vi "Gestion User.vi"(8 "error in (no error)":errorcluster caption="entrée d'erreur (pas d'erreur)", 9 "Fonction":T2(ring), 10 "Commade User":T1) -> (0 "error out":errorcluster caption="sortie d'erreur", 2 "Retour User":T1, 3 "Liste code Operator":string[](array[string]))   [LabVIEW 2020]
uses:
  <vilib>/Utility/config.llb/Config Data RefNum.ctl
  Commande Action Gestion User.ctl
  <vilib>/Utility/config.llb/Read Key (String).vi
  <vilib>/Utility/config.llb/Write Key (String).vi
  <vilib>/Utility/config.llb/NI_LVConfig.lvlib
  Commun VI/Library Commun.lvlib
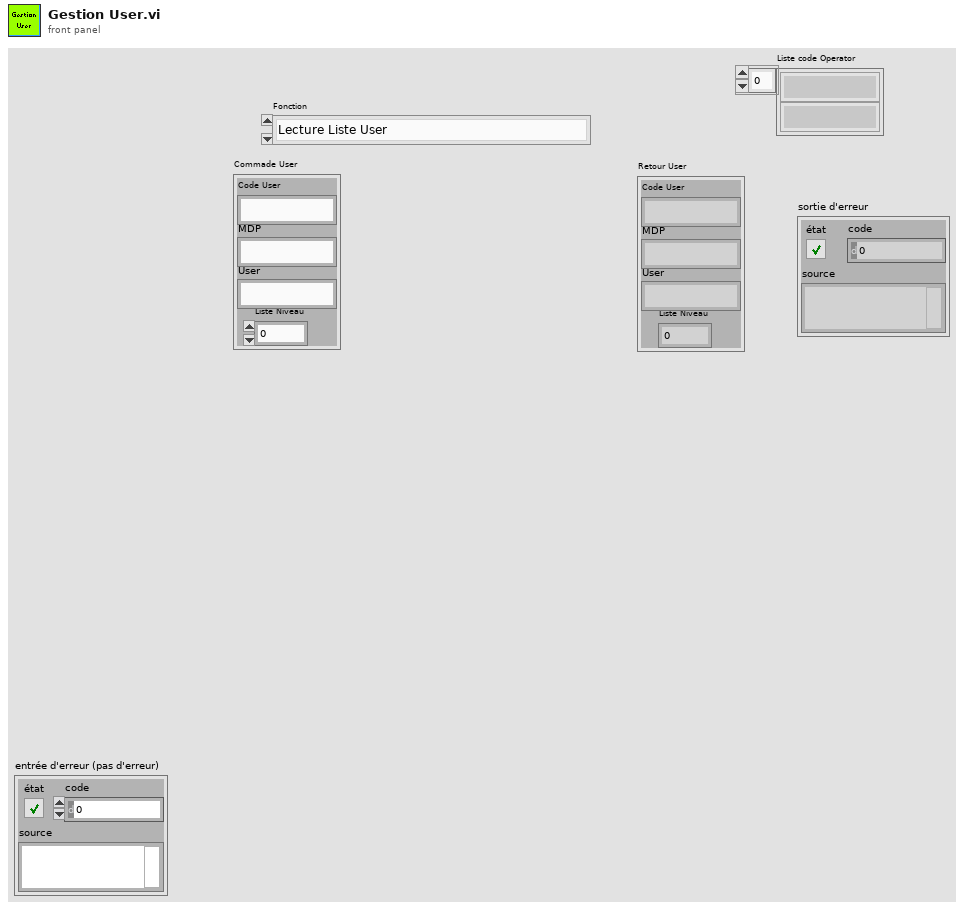
[diagram p1: front panel]
types:
  T1 = cluster{"Code User":string, "MDP":string, "User":string, "Liste Niveau":u16}
  T2 = enum16{"Lecture Liste User", "Lecture User", "Suppression User", "Write User"}
  T3 = cluster{" Section User":string, "Section Grade":string, "Section Password":string}
  T4 = typedef "Commande Action Gestion User.ctl" = enum16{"Ouverture File", "Fermeture File", "Lecture Liste Code User", "Lecture User", "Supression Liste User", "Write User", "Gestion si erreur Decodage"}
  T5 = typedef "NI_LVConfig.lvlib/Config Data RefNum.ctl" = refnum<k1>
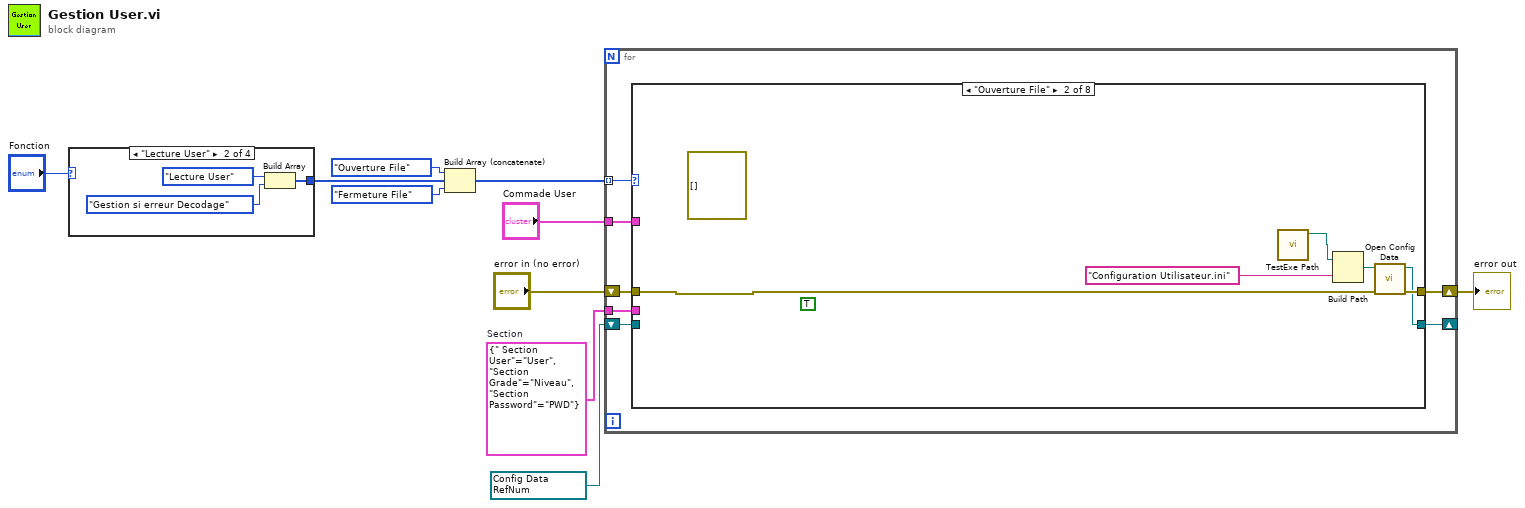
[diagram p0: block diagram]
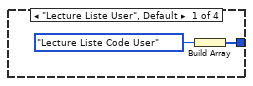
[diagram p2: hidden frame]
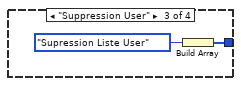
[diagram p3: hidden frame]
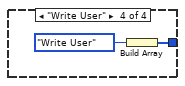
[diagram p4: hidden frame]
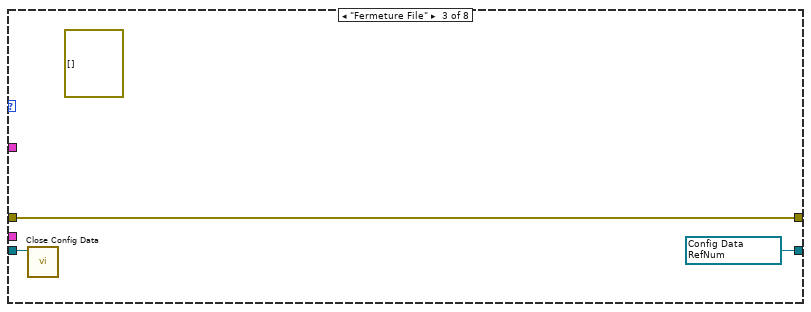
[diagram p6: hidden frame]
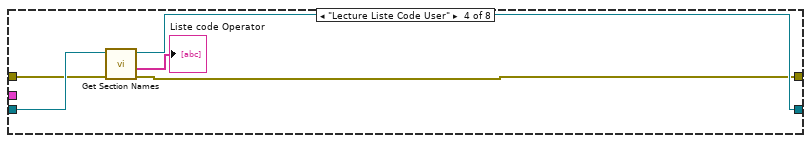
[diagram p7: hidden frame]
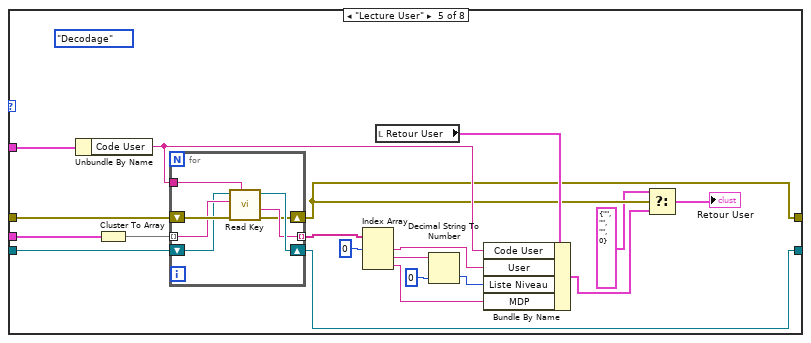
[diagram p8: hidden frame]
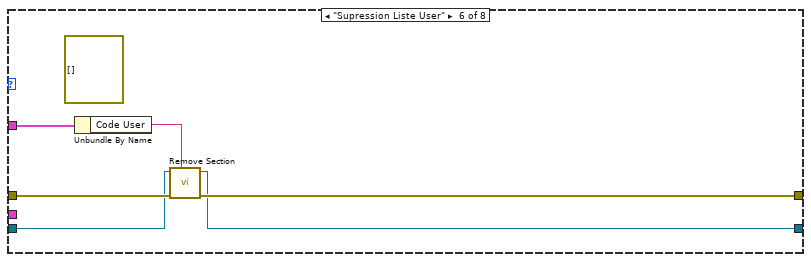
[diagram p9: hidden frame]
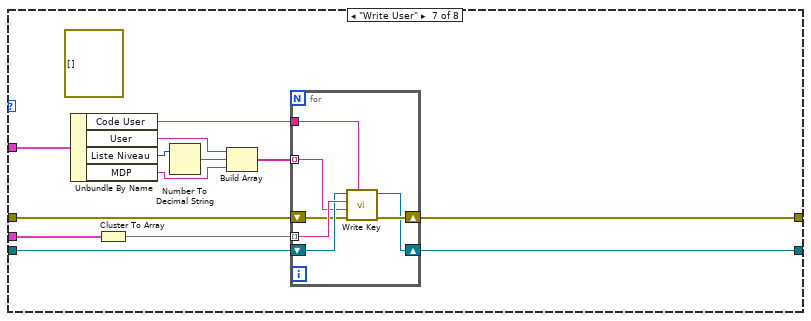
[diagram p10: hidden frame]
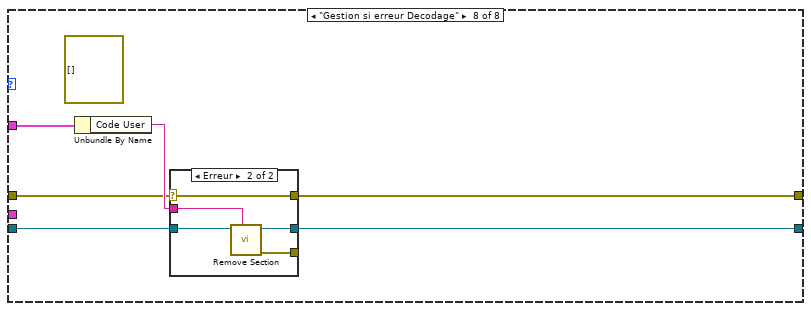
[diagram p11: hidden frame]
diagram:
  w1 = T3 {" Section User"="User", "Section Grade"="Niveau", "Section Password"="PWD"}  # Section
  w8 = T5 refnum items=["config data"] ("refnum")
  n1 = case shown="\"Lecture User\"" "Fonction" {
    tunnel: [w12 w15 w16 w18] -> w5
    frame "Lecture Liste User", Default {
      n2 = Build Array(Commande_Action_Gestion_User."Lecture Liste Code User") -> (w12:T4[])
    }
    frame "Lecture User" {
      n3 = Build Array(Commande_Action_Gestion_User."Lecture User", Commande_Action_Gestion_User."Gestion si erreur Decodage") -> (w15:T4[])
    }
    frame "Suppression User" {
      n4 = Build Array(Commande_Action_Gestion_User."Supression Liste User") -> (w16:T4[])
    }
    frame "Write User" {
      n5 = Build Array(Commande_Action_Gestion_User."Write User") -> (w18:T4[])
    }
  }
  n6 = Build Array (concatenate)(Commande_Action_Gestion_User."Ouverture File", w5, Commande_Action_Gestion_User."Fermeture File") -> (w10:T4[])
  n7 = for {
    tunnel: w10 -> [w22] mode=indexing
    shift-right: [w25] -> w7
    shift-left: "error in (no error)" -> [w26]
    shift-right: [w24] -> _
    shift-left: w8 -> [w23]
    tunnel: "Commade User" -> [w21]
    tunnel: w1 -> [w20]
    n8 = case shown="\"Ouverture File\"" w22 {
      tunnel: w26 -> [w27 w30 w36 w41 w48 w74 w75 w95]
      tunnel: [w27 w32 w36 w38 w46 w73 w82 w99] -> w25
      tunnel: [w28 w31 w35 w40 w59 w71 w80 w98] -> w24
      tunnel: w23 -> [w28 _ w37 w42 w60 w72 w81 w100]
      tunnel: w21 -> [_ _ _ _ w58 w70 w86 w97]
      tunnel: w20 -> [_ _ _ _ w61 _ w87 _]
      frame Default {
      }
      frame "Ouverture File" {
        (unwired) errorcluster[] []
        (unwired) TRUE
        n9 = call "TestExe Path.vi"() -> ("Chemin Actuel"=w29:path)  [unwired: 9 in, 2 out]
        n10 = Build Path(base path=w29, name or relative path="Configuration Utilisateur.ini" ("nom ou chemin relatif")) -> (appended path=w34:path)
        n11 = call <vilib>:"Open Config Data.vi"("error in (no error)"=w30, "configuration file path"=w34) -> ("error out"=w32:errorcluster, "refnum"=w31:T5)  [unwired: 7 in, 1 out]
      }
      frame "Fermeture File" {
        (unwired) errorcluster[] []
        w35 = T5 refnum items=["config data"] ("refnum")
        n12 = call <vilib>:"Close Config Data.vi"("refnum"=w37) -> ()  [unwired: 9 in, 2 out]
      }
      frame "Lecture Liste Code User" {
        n13 = call <vilib>:"Get Section Names.vi"("error in (no error)"=w41, "refnum"=w42) -> ("error out"=w38:errorcluster, "section names"=→"Liste code Operator":string[], "refnum out"=w40:T5)  [unwired: 7 in]
      }
      frame "Lecture User" {
        (unwired) enum16{"Encodage", "Decodage"}."Decodage" ("Fonction")
        n14 = Unbundle By Name(w58) -> ("Code User"=w49:string)
        n15 = Cluster To Array(cluster=w61) -> (array=w57:string[])
        n16 = for {
          tunnel: w49 -> [w67]
          tunnel: w57 -> [w66] mode=indexing
          shift-right: [w62] -> w46
          shift-left: w48 -> [w68]
          shift-right: [w64] -> w59
          shift-left: w60 -> [w65]
          tunnel: [w63] -> w56 mode=indexing
          n17 = call-poly <vilib>:"Read Key.vi"("section"=w67, "error in (no error)"=w68, "key"=w66, "refnum"=w65) -> ("error out"=w62:errorcluster, "value"=w63:string, "refnum out"=w64:T5)  [unwired: 4 in, 1 out]
        }
        n18 = Index Array(array=w56, index #1=0 ("indice")) -> (element #1=w53:string, element #2=w52:string, element #3=w47:string)  [unwired: 2 in]
        n19 = local read "Retour User"() -> (w54:T1)
        n20 = Decimal String To Number(string=w52, default (0L)=u16 0 ("valeur par défaut (0 I32)")) -> (number=w51:u16)  [unwired: 1 in, 1 out]
        n21 = Bundle By Name(cluster=w54, "Code User"=w49, "User"=w53, "Liste Niveau"=w51, "MDP"=w47) -> (w43:T1)
        n22 = Select(t=T1 {"Code User"="", "MDP"="", "User"="", "Liste Niveau"=0} ("Retour User"), s=w46, f=w43) -> (s? t:f=→"Retour User":T1)
      }
      frame "Supression Liste User" {
        (unwired) errorcluster[] []
        n23 = Unbundle By Name(w70) -> ("Code User"=w69:string)
        n24 = call <vilib>:"Remove Section.vi"("section"=w69, "error in (no error)"=w74, "refnum"=w72) -> ("error out"=w73:errorcluster, "refnum out"=w71:T5)  [unwired: 6 in, 1 out]
      }
      frame "Write User" {
        (unwired) errorcluster[] []
        n25 = Unbundle By Name(w86) -> ("Code User"=w77:string, "User"=w85:string, "Liste Niveau"=w84:u16, "MDP"=w76:string)
        n26 = Cluster To Array(cluster=w87) -> (array=w78:string[])
        n27 = Number To Decimal String(number=w84) -> (decimal integer string=w83:string)  [unwired: 1 in]
        n28 = Build Array(w85, w83, w76) -> (w79:string[])
        n29 = for {
          shift-right: [w94] -> w82
          shift-left: w75 -> [w88]
          shift-right: [w91] -> w80
          shift-left: w81 -> [w92]
          tunnel: w79 -> [w90] mode=indexing
          tunnel: w78 -> [w93] mode=indexing
          tunnel: w77 -> [w89]
          n30 = call-poly <vilib>:"Write Key.vi"("section"=w89, "error in (no error)"=w88, "value"=w90, "key"=w93, "refnum"=w92) -> ("error out"=w94:errorcluster, "refnum out"=w91:T5)  [unwired: 4 in, 1 out]
        }
      }
      frame "Gestion si erreur Decodage" {
        (unwired) errorcluster[] []
        n31 = Unbundle By Name(w97) -> ("Code User"=w96:string)
        n32 = case shown="Erreur" w95 {
          selector: w95 -> [w102 w104]
          tunnel: w100 -> [w101 w107]
          tunnel: [w102 w104] -> w99
          tunnel: [w101 w106] -> w98
          tunnel: w96 -> [_ w105]
          tunnel: [_ w103] -> _
          frame No Error {
          }
          frame Error {
            n33 = call <vilib>:"Remove Section.vi"("section"=w105, "refnum"=w107) -> ("error out"=w103:errorcluster, "refnum out"=w106:T5)  [unwired: 7 in, 1 out]
          }
        }
      }
    }
  }
  "error out" <- w7
